vi "HK Write Value.vi"(7 "Timestamp":timestamp, 8 "error in (no error)":errorcluster, 9 "Value":dbl, 10 "Channel Name":string, 11 "HK Channel in":refnum<class "HK Table.lvclass">) -> (0 "error out":errorcluster, 1 "value":T1, 2 "Channel Name dup":string, 3 "HK Channel out":refnum<class "HK Table.lvclass">, 4 "Alarm Status":T2)   [LabVIEW 2024, in "HK Table.lvclass"]
uses:
  HK Table.lvclass
  HK Alarms/HK Alarm enum Status.ctl
  HK Current Value Table Element.ctl
  HK Table.lvclass/HK Table.ctl
  HK Item/HK Item.lvclass
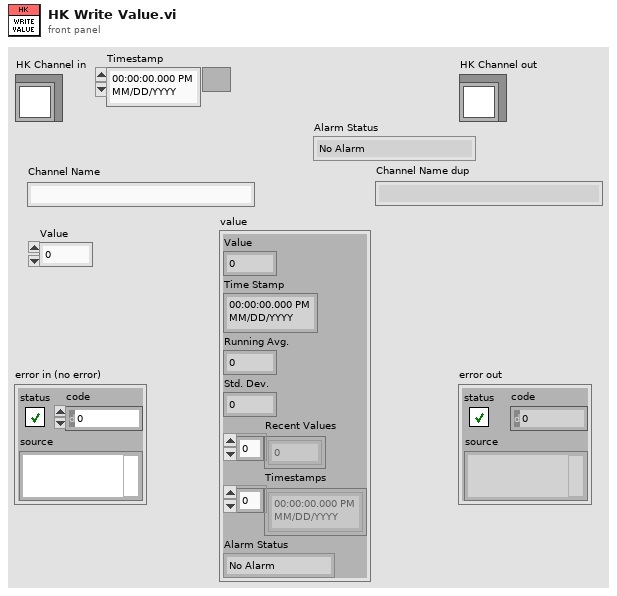
[diagram p1: front panel]
types:
  T1 = typedef "HK Table.lvclass/HK Current Value Table Element.ctl" = cluster{"Value":dbl, "Time Stamp":timestamp, "Running Avg.":dbl, "Std. Dev.":dbl, "Recent Values":dbl[], "Timestamps":timestamp[], "Alarm Status":T2}
  T2 = typedef "HK Item.lvclass/HK Alarm enum Status.ctl" = enum16{"No Alarm", "Red Low", "Red High", "Yellow Low", "Yellow High"}
  T3 = typedef "HK Table.lvclass/HK Current Value Table Settings.ctl" = cluster{"Running Avg Elements":i32, "Max Age":dbl}
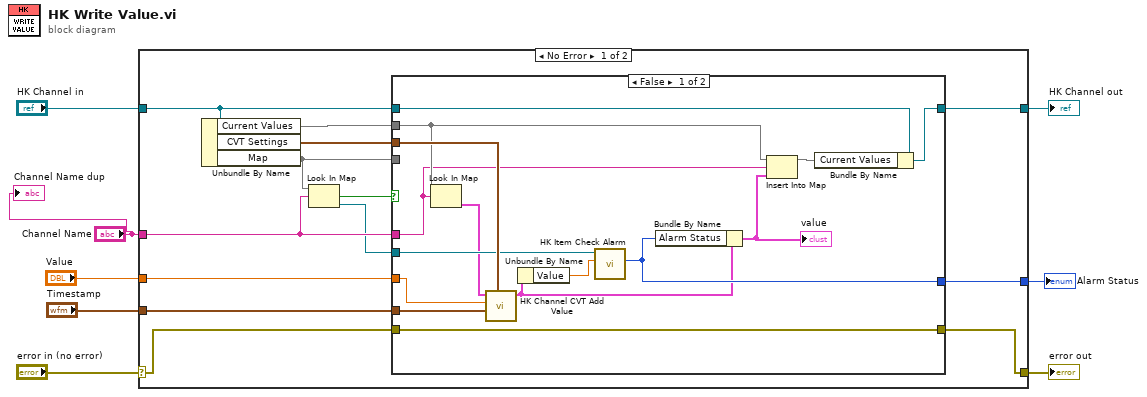
[diagram p0: block diagram]
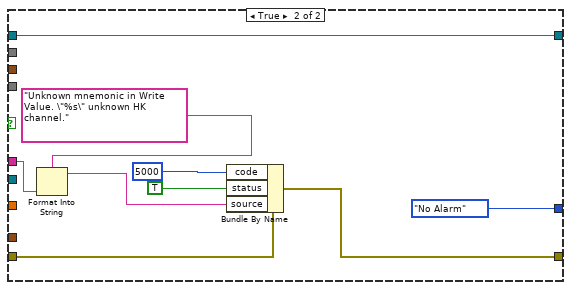
[diagram p2: hidden frame]
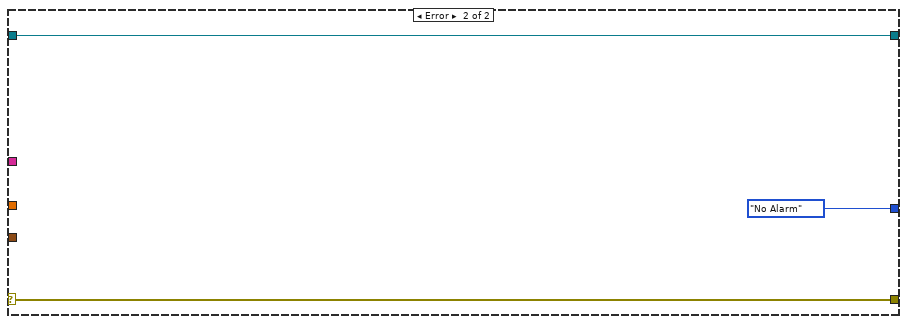
[diagram p3: hidden frame]
diagram:
  n1 = case shown="No Error" "error in (no error)" {
    selector: "error in (no error)" -> [w14 w48]
    tunnel: [w13 w48] -> w7
    tunnel: [w16 w47] -> w5
    tunnel: "HK Channel in" -> [w15 w47]
    tunnel: "Channel Name" -> [w19 _]
    tunnel: "Value" -> [w17 _]
    tunnel: [w10 HK_Alarm_enum_Status."No Alarm" ("Alarm Status")] -> w2
    tunnel: "Timestamp" -> [w9 _]
    frame No Error {
      n2 = Unbundle By Name(w15) -> ("Current Values"=w11:map{string, T1}, "CVT Settings"=w12:T3, "Map"=w20:map{string, refnum<class "HK Item.lvclass">})
      n3 = Look In Map(map=w20, key=w19) -> (key not found?=w21:bool, value=w18:refnum<class "HK Item.lvclass">)  [unwired: 1 in]
      n4 = case shown="False" w21 {
        tunnel: w20 -> [_ _]
        tunnel: w19 -> [w22 w41]
        tunnel: w18 -> [w27 _]
        tunnel: w17 -> [w30 _]
        tunnel: w15 -> [w36 w45]
        tunnel: [w34 w45] -> w16
        tunnel: w14 -> [w33 w40]
        tunnel: [w33 w38] -> w13
        tunnel: w12 -> [w32 _]
        tunnel: w11 -> [w23 _]
        tunnel: [w29 HK_Alarm_enum_Status."No Alarm" ("Alarm Status")] -> w10
        tunnel: w9 -> [w28 _]
        frame False {
          n5 = Look In Map(map=w23, key=w22) -> (value=w26:T1)  [unwired: 1 in, 1 out]
          n6 = call "HK Channel CVT Add Value.vi"("CVT Settings"=w32, "Timestamp"=w28, "New Value"=w30, "Current Value"=w26) -> ("Current Value out"=w24:T1)  [unwired: 6 in, 1 out]
          n7 = Unbundle By Name(w24) -> ("Value"=w25:dbl)
          n8 = call-dynamic "HK Item Check Alarm.vi"("Value"=w25, "HK Item in"=w27) -> ("Alarm Status"=w29:T2)  [unwired: 7 in, 2 out]
          n9 = Bundle By Name(cluster=w24, "Alarm Status"=w29) -> (w31:T1)
          "value" <- w31
          n10 = Insert Into Map(map in=w23, key=w22, value=w31) -> (map out=w35:map{string, T1})  [unwired: 2 out]
          n11 = Bundle By Name(cluster=w36, "Current Values"=w35) -> (w34:refnum<class "HK Table.lvclass">)
        }
        frame True {
          n12 = Format Into String(format string="Unknown mnemonic in Write Value. \"%s\" unknown HK channel.", w41) -> (resulting string=w42:string)  [unwired: 2 in, 1 out]
          n13 = Bundle By Name(cluster=w40, "code"=5000, "status"=TRUE, "source"=w42) -> (w38:errorcluster)
        }
      }
    }
    frame Error {
    }
  }
  "error out" <- w7
  "HK Channel out" <- w5
  "Alarm Status" <- w2
  "Channel Name dup" <- "Channel Name"
